vi "Zustandsfehlerinformation.vi"(6 "Aktionen":T1, 10 "String":string) -> (2 "String":string)   [LabVIEW 2020, in "AK-Schnittstelle.lvlib"]
uses:
  AK-Schnittstelle.lvlib
  Aktionen Zustandsfehlerinformation.ctl
  Aktionen Stoernummern pruefen.ctl
  Stoerungen/Stoerungen.lvlib
  Stoerungen/FGV Stoerung aufnehmen Aktion.ctl
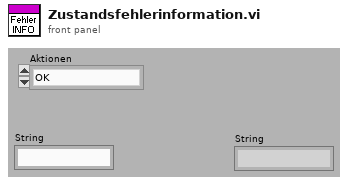
[diagram p1: front panel]
types:
  T1 = typedef "AK-Schnittstelle.lvlib/Aktionen Zustandsfehlerinformation.ctl" = enum16{"OK", "Offline", "Busy", "Syntax Error", "Datenfehler"}
  T2 = typedef "AK-Schnittstelle.lvlib/Aktionen Stoernummern pruefen.ctl" = enum16{"lesen", "prüfen"}
  T3 = typedef "Stoerungen.lvlib/FGV Stoerung aufnehmen Aktion.ctl" = enum16{"Initialisieren", "Schreiben", "Lesen", "Quittieren", "quit. löschen"}
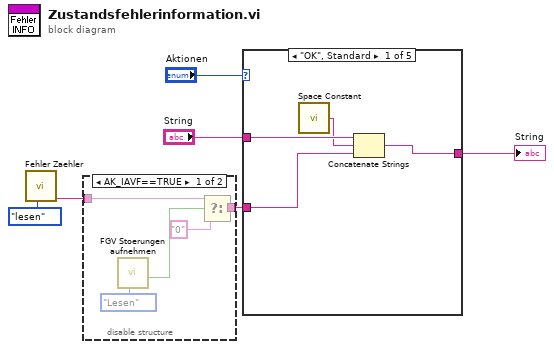
[diagram p0: block diagram]
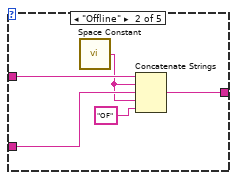
[diagram p3: hidden frame]
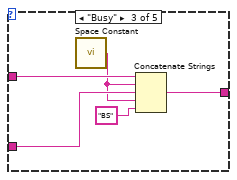
[diagram p4: hidden frame]
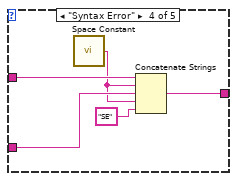
[diagram p5: hidden frame]
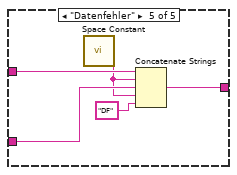
[diagram p6: hidden frame]
diagram:
  n1 = call "Fehler Zaehler.vi"("Aktionen"=Aktionen_Stoernummern_pruefen."lesen") -> ("Fehlerzähler"=w1:string)  [unwired: 7 in, 3 out]
  n2 = disable-structure shown="AK_IAVF==TRUE" {
    disable-tunnel: [w10 w12] -> w2
    disable-tunnel: w1 -> [w9 w12]
    frame condition #0 {
      n3 = call "FGV Stoerungen aufnehmen.vi"("FGV Störung aufnehmen Aktion"=FGV_Stoerung_aufnehmen_Aktion."Lesen") -> ("abschalten"=w8:bool)  [unwired: 7 in, 3 out]
      n4 = Select(t=w9, s=w8, f="0") -> (s? t:f=w10:string)
    }
    frame condition #1 (active) {
    }
  }
  n5 = case shown="\"OK\", Standard" "Aktionen" {
    tunnel: [w16 w21 w26 w31 w36] -> w6
    tunnel: "String" -> [w15 w20 w25 w30 w35]
    tunnel: w2 -> [w14 w18 w23 w28 w33]
    frame "OK", Default {
      n6 = call <vilib>:"Space Constant.vi"() -> ("String"=w13:string)
      n7 = Concatenate Strings(w15, w13, w14) -> (w16:string)
    }
    frame "Offline" {
      n8 = call <vilib>:"Space Constant.vi"() -> ("String"=w17:string)
      n9 = Concatenate Strings(w20, w17, w18, w17, "OF" ("String")) -> (w21:string)
    }
    frame "Busy" {
      n10 = call <vilib>:"Space Constant.vi"() -> ("String"=w22:string)
      n11 = Concatenate Strings(w25, w22, w23, w22, "BS" ("String")) -> (w26:string)
    }
    frame "Syntax Error" {
      n12 = call <vilib>:"Space Constant.vi"() -> ("String"=w27:string)
      n13 = Concatenate Strings(w30, w27, w28, w27, "SE" ("String")) -> (w31:string)
    }
    frame "Datenfehler" {
      n14 = call <vilib>:"Space Constant.vi"() -> ("String"=w32:string)
      n15 = Concatenate Strings(w35, w32, w33, w32, "DF" ("String")) -> (w36:string)
    }
  }
  "String" <- w6
